vi "CTRE_Create_Gearbox.vi"   [LabVIEW 2016]
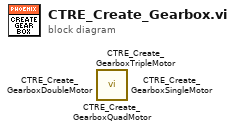
[diagram p0: block diagram]
diagram:
  n1 = call <vilib>:"CTRE_Create_GearboxQuadMotor.vi"() -> ()  [unwired: 11 in, 1 out]
  n2 = call <vilib>:"CTRE_Create_GearboxTripleMotor.vi"() -> ()  [unwired: 11 in, 1 out]
  n3 = call <vilib>:"CTRE_Create_GearboxDoubleMotor.vi"() -> ()  [unwired: 11 in, 1 out]
  n4 = call <vilib>:"CTRE_Create_GearboxSingleMotor.vi"() -> ()  [unwired: 11 in, 1 out]
